vi "Initilaize Sinks.vi"(8 "error in (no error)":errorcluster, 11 "Event Source in":refnum<class "Event Source.lvclass">) -> (0 "error out":errorcluster, 3 "Event Source out":refnum<class "Event Source.lvclass">)   [LabVIEW 2016, in "Event Source.lvlib" / "Event Source.lvclass"]
doc: "This dynamic dispatch VI has to be overriden by the concrete Souce Actor subclasses in order to initilaize the sinks that are going to register for events"
uses:
  Event Source.lvclass
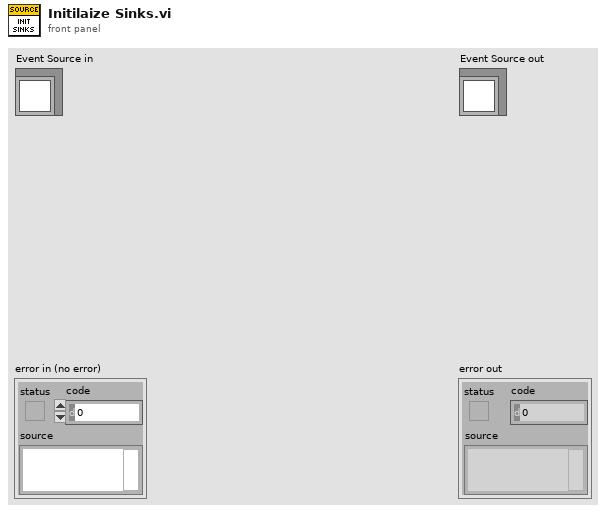
[diagram p1: front panel]
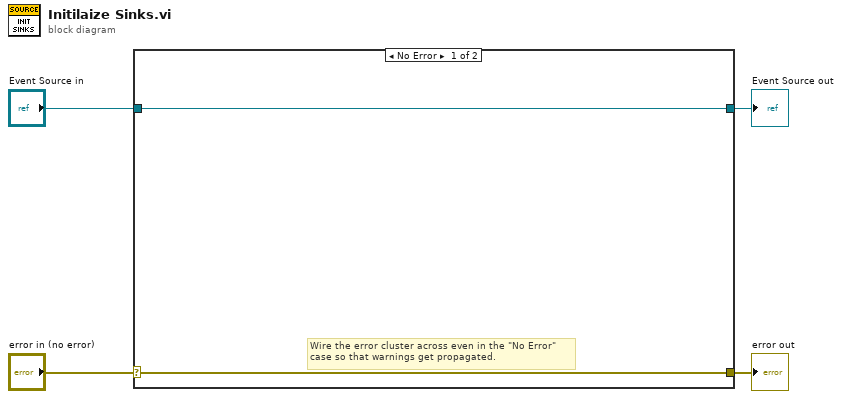
[diagram p0: block diagram]
diagram:
  n1 = case shown="No Error" "error in (no error)" {
    selector: "error in (no error)" -> [w5 w8]
    tunnel: [w5 w8] -> w3
    tunnel: [w6 w7] -> w1
    tunnel: "Event Source in" -> [w6 w7]
    frame No Error {
      # "Wire the error cluster across even in the \"No Error\"\ncase so that warnings get propagated."
    }
    frame Error {
    }
  }
  "error out" <- w3
  "Event Source out" <- w1
